vi "for_v0_v4.vi"() -> ()   [LabVIEW 2010]
panel:
  in  "stop":bool
  in  "Nr_max":u8(slide)=44 scale=0.0..255.0
  out "Numeric":dbl=12.0
  out "Array":bool[](array[boolean])=[FALSE, FALSE, FALSE, FALSE, TRUE, TRUE, FALSE, FALSE]
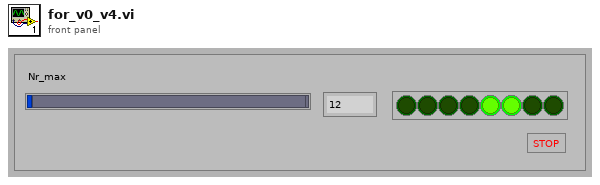
[diagram p1: front panel]
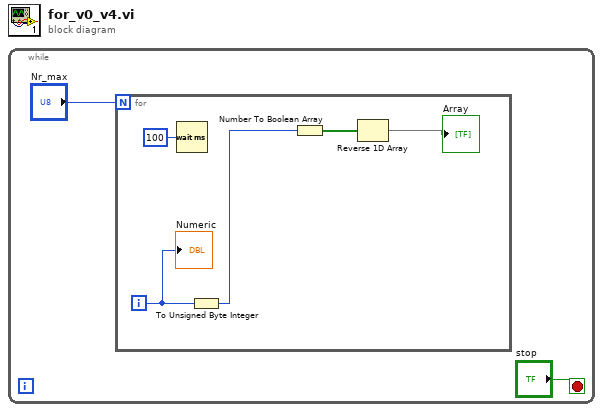
[diagram p0: block diagram]
diagram:
  n1 = while {
    stop <- "stop" stop-if-true
    n2 = for {
      N: "Nr_max" -> [_]
      i -> [w3]
      n3 = Wait (ms)(milliseconds to wait=u32 100) -> ()  [unwired: 1 out]
      n4 = To Unsigned Byte Integer(number=w3) -> (unsigned 8bit integer=w4:u8)
      n5 = Number To Boolean Array(number=w4) -> (Boolean array=w7:bool[])
      n6 = Reverse 1D Array(array=w7) -> (reversed array=→"Array":bool[])
      "Numeric" <- w3
    }
  }
